vi "test Data Types.vi"(8 "error in (no error)":errorcluster, 11 "TestCase in":refnum<class "BNR.lvclass">) -> (0 "error out":errorcluster, 3 "TestCase out":refnum<class "BNR.lvclass">)   [LabVIEW 2020, in "BNR.lvclass"]
uses:
  BNR.lvclass
  ea4660e2-e94a-4730-92e4-4a979d9ba497.vi
  dd848d0f-3c36-47ac-a1a5-bdec4e557583.vi
  8853a246-4140-4473-a418-672ac39e676d.vi
  70a56a29-7605-4fb7-a3c2-9569d1e6a598.vi
  8bc1e205-e619-4779-98f3-d88ede699e43.vi
  0ab31b35-db84-45ff-bc08-0ce488ab4d39.vi
  d9da05b8-8c4b-432a-812e-18e8cf1e7732.vi
  e875d667-e5ee-45ee-93e8-1ede48a590f4.vi
  c99423fd-604f-478d-bbad-01e32088edde.vi
  7e27276a-05e4-4bcc-bc7a-cb86725880cf.vi
  e44283f0-00c1-482d-9767-faa7a6297267.vi
  679bdd48-21e9-4857-8799-eae4867f671a.vi
  93659853-5df4-479f-b147-bcd42bc4e5d6.vi
  093b0240-a2ce-4c94-962c-09d44baff142.vi
  19c52a08-f85b-461a-baf2-65c061ff472d.vi
  0aadc548-88a3-48b5-8e87-c47f67ceed28.vi
  60511d20-a68c-4a95-a779-01fd0b81eb24.vi
  ea4660e2-e94a-4730-92e4-4a979d9ba497.vi/9377bb8f-44b5-4a8f-87f1-966fd5a9edcc.vi
  dd848d0f-3c36-47ac-a1a5-bdec4e557583.vi/9377bb8f-44b5-4a8f-87f1-966fd5a9edcc.vi
  8853a246-4140-4473-a418-672ac39e676d.vi/16a2565b-3c16-407b-a626-9da2a3da432e.vi
  70a56a29-7605-4fb7-a3c2-9569d1e6a598.vi/9377bb8f-44b5-4a8f-87f1-966fd5a9edcc.vi
  8bc1e205-e619-4779-98f3-d88ede699e43.vi/16a2565b-3c16-407b-a626-9da2a3da432e.vi
  0ab31b35-db84-45ff-bc08-0ce488ab4d39.vi/9377bb8f-44b5-4a8f-87f1-966fd5a9edcc.vi
  d9da05b8-8c4b-432a-812e-18e8cf1e7732.vi/16a2565b-3c16-407b-a626-9da2a3da432e.vi
  e875d667-e5ee-45ee-93e8-1ede48a590f4.vi/9377bb8f-44b5-4a8f-87f1-966fd5a9edcc.vi
  c99423fd-604f-478d-bbad-01e32088edde.vi/16a2565b-3c16-407b-a626-9da2a3da432e.vi
  7e27276a-05e4-4bcc-bc7a-cb86725880cf.vi/9377bb8f-44b5-4a8f-87f1-966fd5a9edcc.vi
  e44283f0-00c1-482d-9767-faa7a6297267.vi/16a2565b-3c16-407b-a626-9da2a3da432e.vi
  679bdd48-21e9-4857-8799-eae4867f671a.vi/9377bb8f-44b5-4a8f-87f1-966fd5a9edcc.vi
  93659853-5df4-479f-b147-bcd42bc4e5d6.vi/16a2565b-3c16-407b-a626-9da2a3da432e.vi
  093b0240-a2ce-4c94-962c-09d44baff142.vi/9377bb8f-44b5-4a8f-87f1-966fd5a9edcc.vi
  19c52a08-f85b-461a-baf2-65c061ff472d.vi/16a2565b-3c16-407b-a626-9da2a3da432e.vi
  0aadc548-88a3-48b5-8e87-c47f67ceed28.vi/9377bb8f-44b5-4a8f-87f1-966fd5a9edcc.vi
  60511d20-a68c-4a95-a779-01fd0b81eb24.vi/16a2565b-3c16-407b-a626-9da2a3da432e.vi
  <vilib>/addons/_JKI Toolkits/VI Tester/TestCase.llb/TestCase.lvclass
  C:/Program Files (x86)/National Instruments/LabVIEW 2020/vi.lib/addons/_JKI Toolkits/VI Tester/TestCase.llb/TestCase.lvclass
panel:
  out "BCD encoded value":bool[](array[boolean])
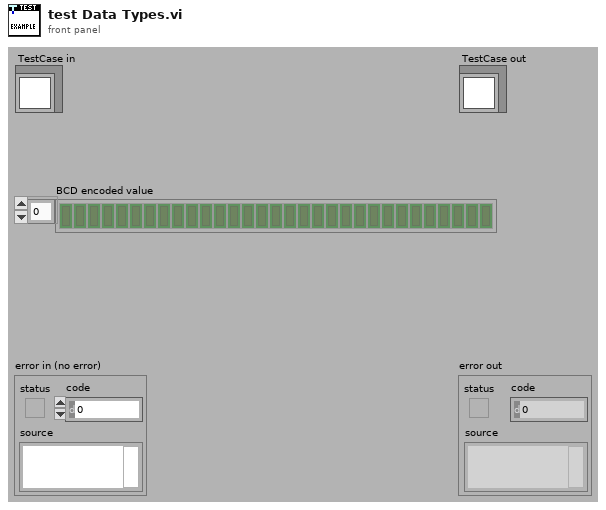
[diagram p1: front panel]
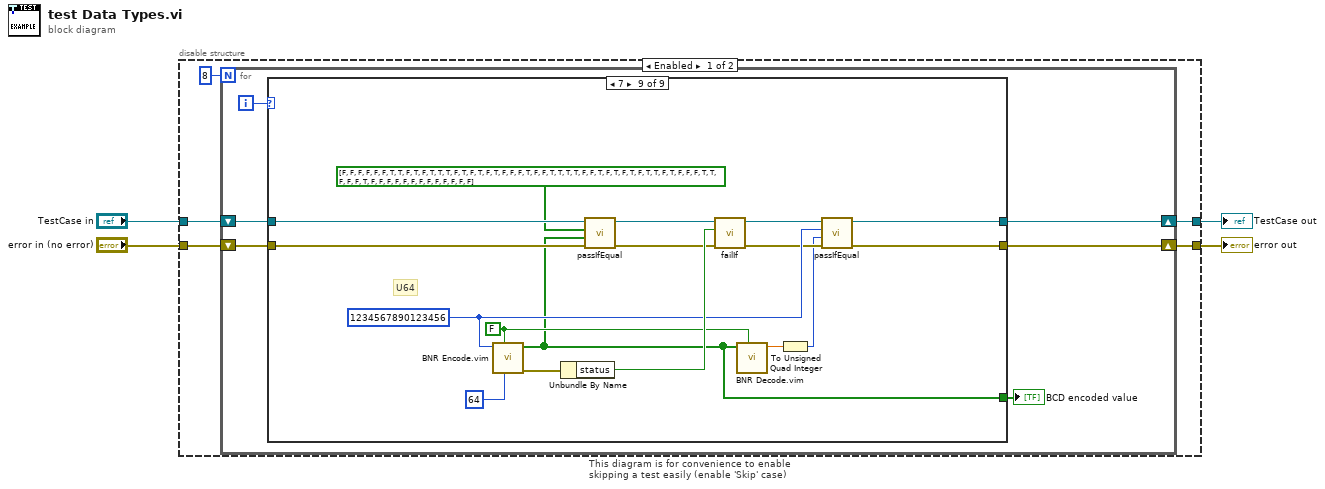
[diagram p0: block diagram]
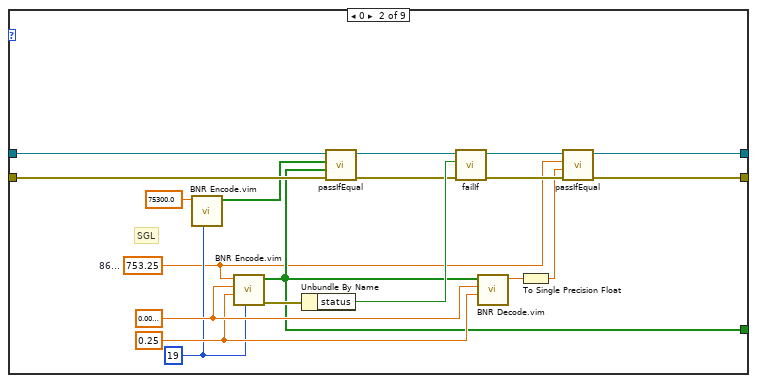
[diagram p3: hidden frame]
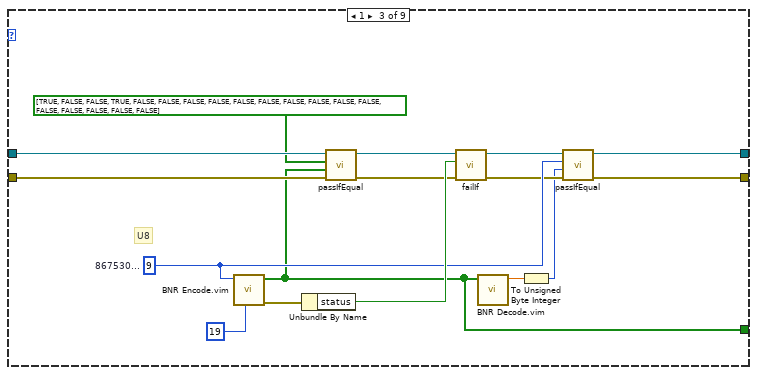
[diagram p4: hidden frame]
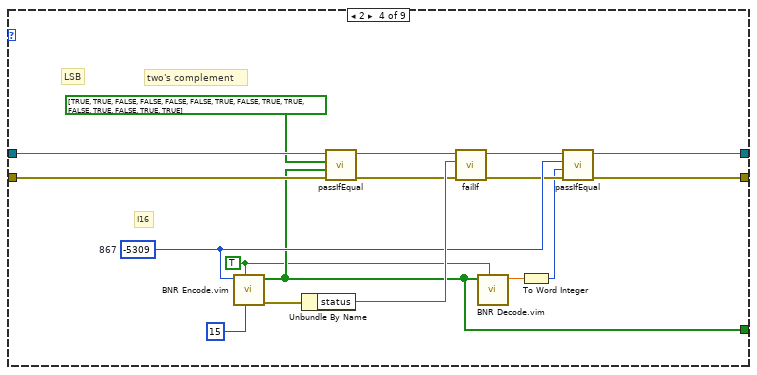
[diagram p5: hidden frame]
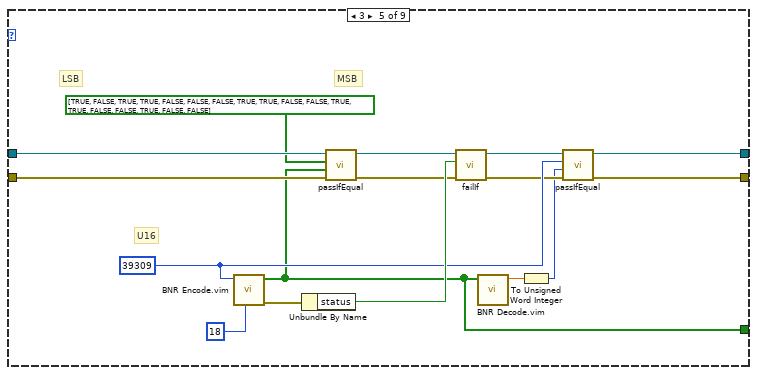
[diagram p6: hidden frame]
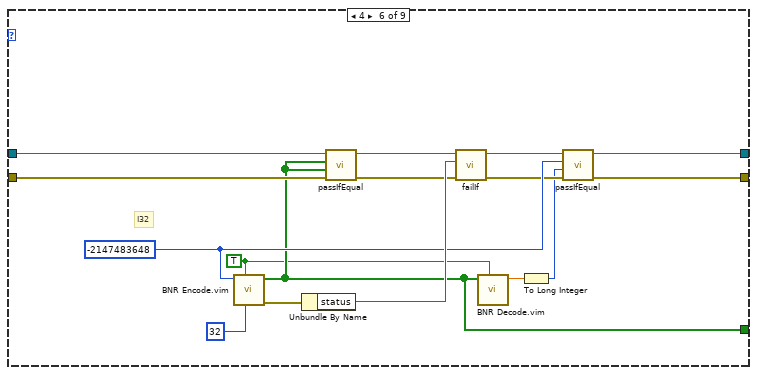
[diagram p7: hidden frame]
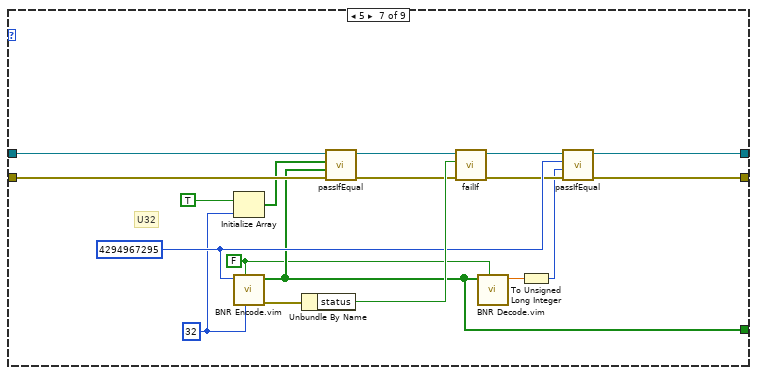
[diagram p8: hidden frame]
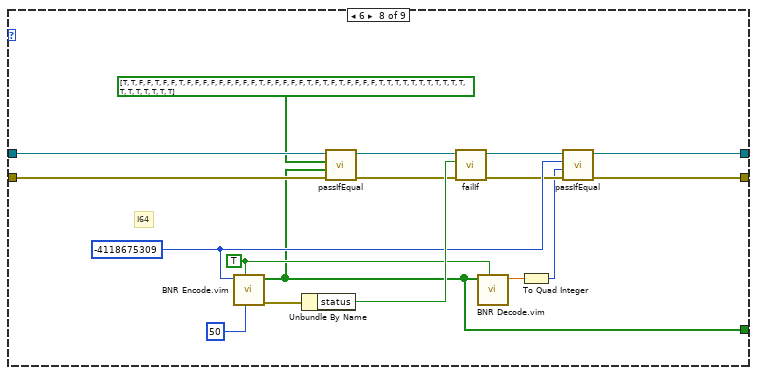
[diagram p9: hidden frame]
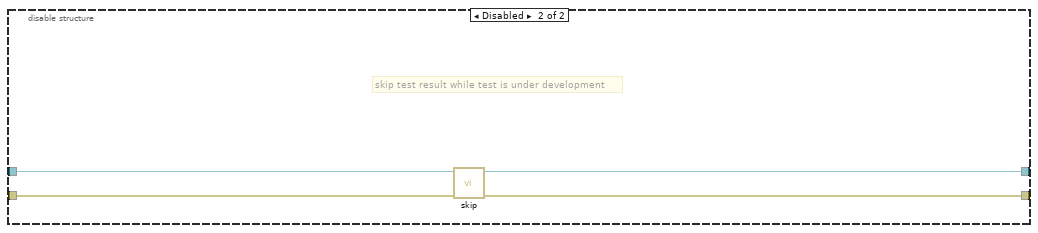
[diagram p10: hidden frame]
diagram:
  n1 = disable-structure "This diagram is for convenience to enable skipping a test easily (enable 'Skip' case)" shown="Enabled" {
    disable-tunnel: "TestCase in" -> [w9 w157]
    disable-tunnel: [w6 w155] -> w3
    disable-tunnel: [w7 w156] -> w1
    disable-tunnel: "error in (no error)" -> [w8 w154]
    frame Enabled {
      n2 = for {
        N: 8 -> [_]
        shift-right: [w12] -> w6
        shift-left: w9 -> [w15]
        shift-right: [w13] -> w7
        shift-left: w8 -> [w14]
        i -> [w11]
        n3 = case shown="7" w11 {
          tunnel: w15 -> [w17 w35 w50 w67 w83 w99 w118 w134 w151]
          tunnel: w14 -> [w16 w34 w49 w66 w82 w98 w117 w133 w150]
          tunnel: [w16 w25 w40 w57 w73 w90 w109 w125 w142] -> w13
          tunnel: [w17 w24 w39 w56 w72 w89 w108 w124 w141] -> w12
          tunnel: [_ w23 w37 w54 w70 w87 w106 w120 w137] -> w10
          frame Default {
          }
          frame 0 {
            w30 = sgl 0.25 ("scale multiplier")
            w31 = sgl 0.01 ("scale multiplier")
            w22 = 19 ("data size (bits)")
            w19 = sgl 753.25  # 86...
            # "SGL"
            n4 = call "BNR Encode.vim"("data size (bits)"=w22, "value"=sgl 75300.0) -> ("BNR encoded value"=w20:bool[])  [unwired: 8 in, 1 out]
            n5 = call "BNR Encode.vim"("data size (bits)"=w22, "scale offset"=w30, "scale multiplier"=w31, "value"=w19) -> ("error out"=w33:errorcluster, "BNR encoded value"=w23:bool[])  [unwired: 6 in]
            n6 = Unbundle By Name(w33) -> ("status"=w32:bool)
            n7 = call-dynamic "passIfEqual.vi"("error in (no error)"=w34, "y"=w23, "x"=w20, "TestCase in"=w35) -> ("error out"=w28:errorcluster, "TestCase out"=w29:refnum<class "BNR.lvclass">)  [unwired: 6 in]
            n8 = call-dynamic "failIf.vi"("error in (no error)"=w28, "fail"=w32, "TestCase in"=w29) -> ("error out"=w26:errorcluster, "TestCase out"=w27:refnum<class "BNR.lvclass">)  [unwired: 7 in]
            n9 = call "BNR Decode.vim"("scale offset"=w30, "scale multiplier"=w31, "BNR encoded value"=w23) -> ("value"=w36:dbl)  [unwired: 8 in]
            n10 = To Single Precision Float(number=w36) -> (single precision float=w18:sgl)
            n11 = call-dynamic "passIfEqual.vi"("error in (no error)"=w26, "y"=w18, "x"=w19, "TestCase in"=w27) -> ("error out"=w25:errorcluster, "TestCase out"=w24:refnum<class "BNR.lvclass">)  [unwired: 6 in]
          }
          frame 1 {
            w45 = u8 9  # 867530...
            # "U8"
            n12 = call "BNR Encode.vim"("data size (bits)"=19, "value"=w45) -> ("error out"=w47:errorcluster, "BNR encoded value"=w37:bool[])  [unwired: 8 in]
            n13 = Unbundle By Name(w47) -> ("status"=w46:bool)
            n14 = call-dynamic "passIfEqual.vi"("error in (no error)"=w49, "y"=w37, "x"=bool[] [TRUE, FALSE, FALSE, TRUE, FALSE, FALSE, FALSE, FALSE, FALSE, FALSE, FALSE, FALSE, FALSE, FALSE, FALSE, FALSE, FALSE, FALSE, FALSE] ("BCD encoded value"), "TestCase in"=w50) -> ("error out"=w43:errorcluster, "TestCase out"=w44:refnum<class "BNR.lvclass">)  [unwired: 6 in]
            n15 = call-dynamic "failIf.vi"("error in (no error)"=w43, "fail"=w46, "TestCase in"=w44) -> ("error out"=w41:errorcluster, "TestCase out"=w42:refnum<class "BNR.lvclass">)  [unwired: 7 in]
            n16 = call "BNR Decode.vim"("BNR encoded value"=w37) -> ("value"=w51:dbl)  [unwired: 10 in]
            n17 = To Unsigned Byte Integer(number=w51) -> (unsigned 8bit integer=w38:u8)
            n18 = call-dynamic "passIfEqual.vi"("error in (no error)"=w41, "y"=w38, "x"=w45, "TestCase in"=w42) -> ("error out"=w40:errorcluster, "TestCase out"=w39:refnum<class "BNR.lvclass">)  [unwired: 6 in]
          }
          frame 2 {
            w53 = TRUE ("signed")
            w62 = i16 -5309  # 867
            # "two's complement"
            # "LSB"
            # "I16"
            n19 = call "BNR Encode.vim"("data size (bits)"=15, "signed"=w53, "value"=w62) -> ("error out"=w64:errorcluster, "BNR encoded value"=w54:bool[])  [unwired: 7 in]
            n20 = Unbundle By Name(w64) -> ("status"=w63:bool)
            n21 = call-dynamic "passIfEqual.vi"("error in (no error)"=w66, "y"=w54, "x"=bool[] [TRUE, TRUE, FALSE, FALSE, FALSE, FALSE, TRUE, FALSE, TRUE, TRUE, FALSE, TRUE, FALSE, TRUE, TRUE] ("BCD encoded value"), "TestCase in"=w67) -> ("error out"=w60:errorcluster, "TestCase out"=w61:refnum<class "BNR.lvclass">)  [unwired: 6 in]
            n22 = call-dynamic "failIf.vi"("error in (no error)"=w60, "fail"=w63, "TestCase in"=w61) -> ("error out"=w58:errorcluster, "TestCase out"=w59:refnum<class "BNR.lvclass">)  [unwired: 7 in]
            n23 = call "BNR Decode.vim"("signed"=w53, "BNR encoded value"=w54) -> ("value"=w68:dbl)  [unwired: 9 in]
            n24 = To Word Integer(number=w68) -> (16bit integer=w55:i16)
            n25 = call-dynamic "passIfEqual.vi"("error in (no error)"=w58, "y"=w55, "x"=w62, "TestCase in"=w59) -> ("error out"=w57:errorcluster, "TestCase out"=w56:refnum<class "BNR.lvclass">)  [unwired: 6 in]
          }
          frame 3 {
            w78 = u16 39309 ("867...")
            # "U16"
            # "MSB"
            # "LSB"
            n26 = call "BNR Encode.vim"("data size (bits)"=18, "value"=w78) -> ("error out"=w80:errorcluster, "BNR encoded value"=w70:bool[])  [unwired: 8 in]
            n27 = Unbundle By Name(w80) -> ("status"=w79:bool)
            n28 = call-dynamic "passIfEqual.vi"("error in (no error)"=w82, "y"=w70, "x"=bool[] [TRUE, FALSE, TRUE, TRUE, FALSE, FALSE, FALSE, TRUE, TRUE, FALSE, FALSE, TRUE, TRUE, FALSE, FALSE, TRUE, FALSE, FALSE] ("BCD encoded value"), "TestCase in"=w83) -> ("error out"=w76:errorcluster, "TestCase out"=w77:refnum<class "BNR.lvclass">)  [unwired: 6 in]
            n29 = call-dynamic "failIf.vi"("error in (no error)"=w76, "fail"=w79, "TestCase in"=w77) -> ("error out"=w74:errorcluster, "TestCase out"=w75:refnum<class "BNR.lvclass">)  [unwired: 7 in]
            n30 = call "BNR Decode.vim"("BNR encoded value"=w70) -> ("value"=w84:dbl)  [unwired: 10 in]
            n31 = To Unsigned Word Integer(number=w84) -> (unsigned 16bit integer=w71:u16)
            n32 = call-dynamic "passIfEqual.vi"("error in (no error)"=w74, "y"=w71, "x"=w78, "TestCase in"=w75) -> ("error out"=w73:errorcluster, "TestCase out"=w72:refnum<class "BNR.lvclass">)  [unwired: 6 in]
          }
          frame 4 {
            w86 = TRUE ("signed")
            w95 = -2147483648 ("867...")
            # "I32"
            n33 = call "BNR Encode.vim"("data size (bits)"=32, "signed"=w86, "value"=w95) -> ("error out"=w97:errorcluster, "BNR encoded value"=w87:bool[])  [unwired: 7 in]
            n34 = Unbundle By Name(w97) -> ("status"=w96:bool)
            n35 = call-dynamic "passIfEqual.vi"("error in (no error)"=w98, "y"=w87, "x"=w87, "TestCase in"=w99) -> ("error out"=w93:errorcluster, "TestCase out"=w94:refnum<class "BNR.lvclass">)  [unwired: 6 in]
            n36 = call-dynamic "failIf.vi"("error in (no error)"=w93, "fail"=w96, "TestCase in"=w94) -> ("error out"=w91:errorcluster, "TestCase out"=w92:refnum<class "BNR.lvclass">)  [unwired: 7 in]
            n37 = call "BNR Decode.vim"("signed"=w86, "BNR encoded value"=w87) -> ("value"=w100:dbl)  [unwired: 9 in]
            n38 = To Long Integer(number=w100) -> (32bit integer=w88:i32)
            n39 = call-dynamic "passIfEqual.vi"("error in (no error)"=w91, "y"=w88, "x"=w95, "TestCase in"=w92) -> ("error out"=w90:errorcluster, "TestCase out"=w89:refnum<class "BNR.lvclass">)  [unwired: 6 in]
          }
          frame 5 {
            w105 = FALSE ("signed")
            w103 = 32 ("data size (bits)")
            w114 = u32 4294967295 ("867...")
            # "U32"
            n40 = Initialize Array(TRUE ("signed"), w103) -> (w102:bool[])
            n41 = call "BNR Encode.vim"("data size (bits)"=w103, "signed"=w105, "value"=w114) -> ("error out"=w116:errorcluster, "BNR encoded value"=w106:bool[])  [unwired: 7 in]
            n42 = Unbundle By Name(w116) -> ("status"=w115:bool)
            n43 = call-dynamic "passIfEqual.vi"("error in (no error)"=w117, "y"=w106, "x"=w102, "TestCase in"=w118) -> ("error out"=w112:errorcluster, "TestCase out"=w113:refnum<class "BNR.lvclass">)  [unwired: 6 in]
            n44 = call-dynamic "failIf.vi"("error in (no error)"=w112, "fail"=w115, "TestCase in"=w113) -> ("error out"=w110:errorcluster, "TestCase out"=w111:refnum<class "BNR.lvclass">)  [unwired: 7 in]
            n45 = call "BNR Decode.vim"("signed"=w105, "BNR encoded value"=w106) -> ("value"=w119:dbl)  [unwired: 9 in]
            n46 = To Unsigned Long Integer(number=w119) -> (unsigned 32bit integer=w107:u32)
            n47 = call-dynamic "passIfEqual.vi"("error in (no error)"=w110, "y"=w107, "x"=w114, "TestCase in"=w111) -> ("error out"=w109:errorcluster, "TestCase out"=w108:refnum<class "BNR.lvclass">)  [unwired: 6 in]
          }
          frame 6 {
            w122 = TRUE ("signed")
            w130 = i64 -4118675309 ("867...")
            # "I64"
            n48 = call "BNR Encode.vim"("data size (bits)"=50, "signed"=w122, "value"=w130) -> ("error out"=w132:errorcluster, "BNR encoded value"=w120:bool[])  [unwired: 7 in]
            n49 = Unbundle By Name(w132) -> ("status"=w131:bool)
            n50 = call-dynamic "passIfEqual.vi"("error in (no error)"=w133, "y"=w120, "x"=bool[] [TRUE, TRUE, FALSE, FALSE, TRUE, FALSE, FALSE, TRUE, FALSE, FALSE, FALSE, FALSE, FALSE, FALSE, FALSE, FALSE, FALSE, TRUE, FALSE, FALSE, FALSE, FALSE, FALSE, TRUE, FALSE, TRUE, FALSE, TRUE, FALSE, FALSE, FALSE, FALSE, TRUE, TRUE, TRUE, TRUE, TRUE, TRUE, TRUE, TRUE, TRUE, TRUE, TRUE, TRUE, TRUE, TRUE, TRUE, TRUE, TRUE, TRUE] ("BCD encoded value"), "TestCase in"=w134) -> ("error out"=w128:errorcluster, "TestCase out"=w129:refnum<class "BNR.lvclass">)  [unwired: 6 in]
            n51 = call-dynamic "failIf.vi"("error in (no error)"=w128, "fail"=w131, "TestCase in"=w129) -> ("error out"=w126:errorcluster, "TestCase out"=w127:refnum<class "BNR.lvclass">)  [unwired: 7 in]
            n52 = call "BNR Decode.vim"("signed"=w122, "BNR encoded value"=w120) -> ("value"=w135:dbl)  [unwired: 9 in]
            n53 = To Quad Integer(1:w135) -> (0:w123:i64)
            n54 = call-dynamic "passIfEqual.vi"("error in (no error)"=w126, "y"=w123, "x"=w130, "TestCase in"=w127) -> ("error out"=w125:errorcluster, "TestCase out"=w124:refnum<class "BNR.lvclass">)  [unwired: 6 in]
          }
          frame 7 {
            w139 = FALSE ("signed")
            w147 = u64 1234567890123456 ("867...")
            # "U64"
            n55 = call "BNR Encode.vim"("data size (bits)"=64, "signed"=w139, "value"=w147) -> ("error out"=w149:errorcluster, "BNR encoded value"=w137:bool[])  [unwired: 7 in]
            n56 = Unbundle By Name(w149) -> ("status"=w148:bool)
            n57 = call-dynamic "passIfEqual.vi"("error in (no error)"=w150, "y"=w137, "x"=bool[] [FALSE, FALSE, FALSE, FALSE, FALSE, FALSE, TRUE, TRUE, FALSE, TRUE, FALSE, TRUE, TRUE, TRUE, FALSE, TRUE, FALSE, TRUE, FALSE, TRUE, FALSE, FALSE, FALSE, TRUE, FALSE, FALSE, TRUE, TRUE, TRUE, TRUE, FALSE, FALSE, TRUE, FALSE, TRUE, FALSE, TRUE, FALSE, TRUE, TRUE, FALSE, TRUE, FALSE, FALSE, FALSE, TRUE, TRUE, FALSE, FALSE, FALSE, TRUE, FALSE, FALSE, FALSE, FALSE, FALSE, FALSE, FALSE, FALSE, FALSE, FALSE, FALSE, FALSE, FALSE] ("BCD encoded value"), "TestCase in"=w151) -> ("error out"=w145:errorcluster, "TestCase out"=w146:refnum<class "BNR.lvclass">)  [unwired: 6 in]
            n58 = call-dynamic "failIf.vi"("error in (no error)"=w145, "fail"=w148, "TestCase in"=w146) -> ("error out"=w143:errorcluster, "TestCase out"=w144:refnum<class "BNR.lvclass">)  [unwired: 7 in]
            n59 = call "BNR Decode.vim"("signed"=w139, "BNR encoded value"=w137) -> ("value"=w152:dbl)  [unwired: 9 in]
            n60 = To Unsigned Quad Integer(1:w152) -> (0:w140:u64)
            n61 = call-dynamic "passIfEqual.vi"("error in (no error)"=w143, "y"=w140, "x"=w147, "TestCase in"=w144) -> ("error out"=w142:errorcluster, "TestCase out"=w141:refnum<class "BNR.lvclass">)  [unwired: 6 in]
          }
        }
        "BCD encoded value" <- w10
      }
    }
    frame Disabled {
      # "skip test result while test is under development"
      n62 = call <vilib>:"skip.vi"("error in (no error)"=w154, "TestCase in"=w157) -> ("error out"=w156:errorcluster, "TestCase out"=w155:refnum<class "BNR.lvclass">)  [unwired: 8 in]
    }
  }
  "error out" <- w1
  "TestCase out" <- w3
